vi "GetIDSN(SubVI).vi"(10 "sn":string) -> (3 "output frame":string)   [LabVIEW 2012]
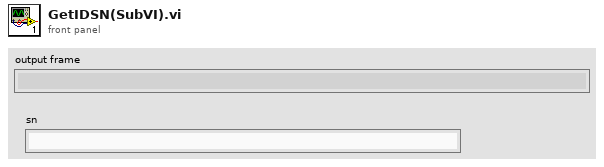
[diagram p1: front panel]
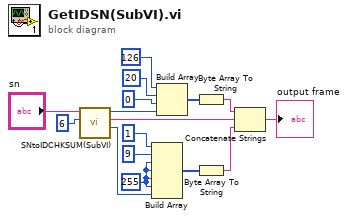
[diagram p0: block diagram]
diagram:
  w2 = u8 255
  n1 = call "SNtoIDCHKSUM(SubVI).vi"("fix cheksum"=u8 6, "input sn"="sn") -> ("output check sum"=w1:u8, "output sn"=w7:string, "output id"=w12:u8)  [unwired: 7 in]
  n2 = Build Array(u8 1, u8 9, w2, w2, w2, w2, w1) -> (w9:u8[])
  n3 = Build Array(u8 126, u8 20, u8 0, w12) -> (w11:u8[])
  n4 = Byte Array To String(unsigned byte array=w11) -> (string=w8:string)
  n5 = Byte Array To String(unsigned byte array=w9) -> (string=w6:string)
  n6 = Concatenate Strings(w8, w7, w6) -> (→"output frame":string)
